vi "Make Floating Point Position.vi"(5 "Floating Point Position (2)":i32=2) -> (6 "Times":dbl)   [LabVIEW 2020, in "Yokogawa GX Series.lvlib"]
doc: "This VI gets the times number of floating point position."
uses:
  <instrlib>/Yokogawa GX Series/Yokogawa GX Series.lvlib
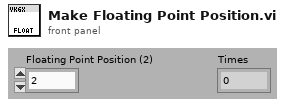
[diagram p1: front panel]
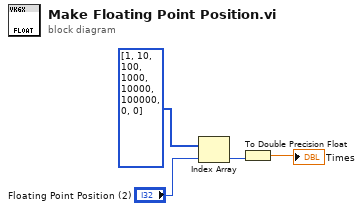
[diagram p0: block diagram]
diagram:
  n1 = Index Array(array=i32[] [1, 10, 100, 1000, 10000, 100000, 0, 0], index="Floating Point Position (2)") -> (element=w2:i32)
  n2 = To Double Precision Float(number=w2) -> (double precision float=→"Times":dbl)
